vi "Nested Alias Unique.vi"(10 "Nested Alias":string, 11 "Dev Actor in":refnum<class "Dev Actor.lvclass">) -> (2 "Nested Alias Unique?":bool)   [LabVIEW 2021, in "Dev Actor.lvlib" / "Dev Actor.lvclass"]
uses:
  Dev Actor.lvclass
  Dev Actor.lvclass/Dev Actor.ctl
  Actor/Queue Actor/Queue Actor.lvclass
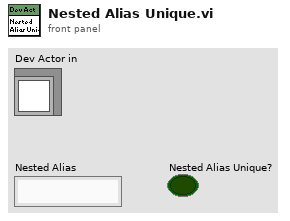
[diagram p1: front panel]
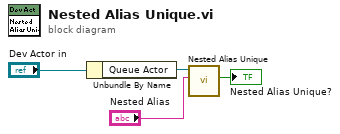
[diagram p0: block diagram]
diagram:
  n1 = Unbundle By Name("Dev Actor in") -> ("Queue Actor"=w3:refnum<class "Queue Actor.lvclass">)
  n2 = call-dynamic "Nested Alias Unique.vi"("Nested Alias"="Nested Alias", "Queue Actor in"=w3) -> ("Nested Alias Unique?"=→"Nested Alias Unique?":bool)  [unwired: 9 in]
